vi "Read Allow Undefined Names.vi"(8 "error in (no error)":errorcluster, 11 "DAQChannelName.lvclass in":refnum<class "DAQChannelName.lvclass">) -> (0 "error out":errorcluster, 2 "AllowUndefNames":bool, 3 "DAQChannelName.lvclass out":refnum<class "DAQChannelName.lvclass">)   [LabVIEW 2015, in "DAQChannelName.lvclass"]
uses:
  DAQChannelName.lvclass
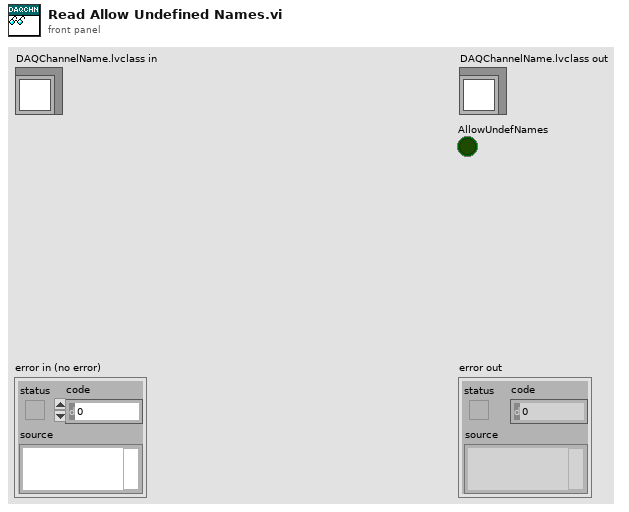
[diagram p1: front panel]
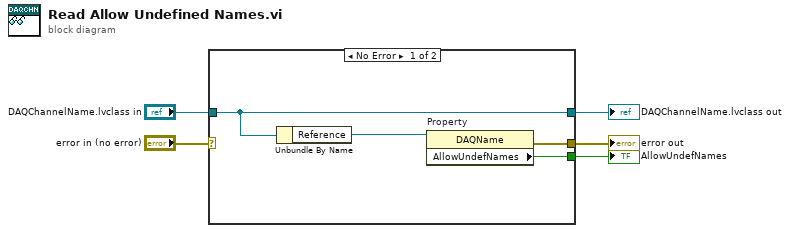
[diagram p0: block diagram]
diagram:
  n1 = case shown="No Error" "error in (no error)" {
    selector: "error in (no error)" -> [_ w11]
    tunnel: [w8 w11] -> w4
    tunnel: [w7 w10] -> w2
    tunnel: "DAQChannelName.lvclass in" -> [w7 w10]
    tunnel: [w9 _] -> w1
    frame No Error {
      n2 = Unbundle By Name(w7) -> ("Reference"=w6:refnum<vi>)
      n3 = property on="Property" class="DAQName"(reference=w6) -> (error out=w8:errorcluster, "AllowUndefNames"=w9:bool)  [unwired: 1 in, 1 out]
    }
    frame Error {
    }
  }
  "error out" <- w4
  "DAQChannelName.lvclass out" <- w2
  "AllowUndefNames" <- w1
